vi "UpdateClassTemplate.vi"(0 "ClassWriterGOOP300In":refnum<class "ClassWriterGOOP300.lvclass">, 1 "LVClassLibraryRef":refnum<vi>, 2 "ProgressBar":refnum<vi>, 5 "error in (no error)":errorcluster) -> (14 "ClassWriterGOOP300Out":refnum<class "ClassWriterGOOP300.lvclass">, 19 "error out":errorcluster)   [LabVIEW 2016, in "ClassWriterGOOP300.lvclass"]
uses:
  <resource>/Framework/Providers/Open_GDS/ClassProviders/Provider_EndevoGOOP300/ClassWriterGOOP300_class/ClassWriterGOOP300.lvclass
  <resource>/Framework/Providers/Open_GDS/ClassProviders/Common/ScriptingFunctions/Scripting.lvclass
  <resource>/Framework/Providers/Open_GDS/ClassProviders/Provider_LvNativeClass/ClassWriterNative_class/ClassWriterNative.lvclass
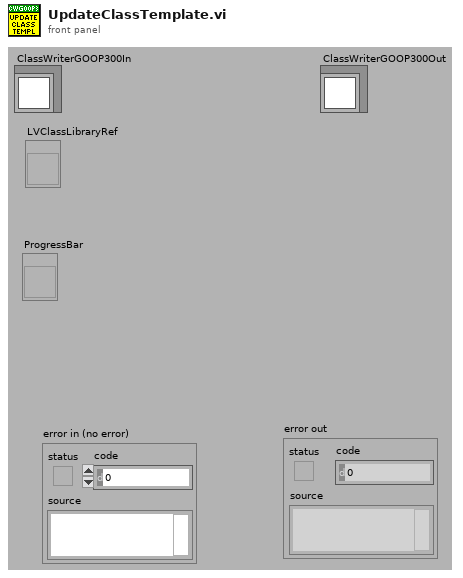
[diagram p1: front panel]
types:
  T1 = cluster{"VIs":refnum<vi>[], "VIRelPath":path[], "Application":refnum<vi>, "TemplateVersions":string, "Create":refnum<vi>, "NewVIIdx":i32}
  T2 = enum32{"invalid lock state", "Not Locked", "Locked (No Password)", "Password-protected"}
  T3 = enum16{"Share clones between instances", "Preallocate clone for each instance"}
  T4 = typedef "Scripting.lvclass/Scripting_PastThroughObjectType.ctl" = cluster{"Object":refnum<vi>, "InsideArray":bool, "PastThroughObjectTypes":T5[], "ObjectType":string, "ObjectData":string}
  T5 = typedef "Scripting_ObjectType.ctl" = cluster{"ObjectType":string, "ObjectName":string, "ObjectTerminalName":string}
  T6 = typedef "GDSLvCLass_ClassSettingsType.ctl" = cluster{"ClassProviderName":string, "ClassTemplateUsed":string, "ClassTemplateVersion":string, "ClassDescription":string, "PlugIns":T7[], "ConnectorPanePattern":string}
  T7 = typedef "GDSLvClass_PlugIn.ctl" = cluster{"Type":T8, "ID":string, "Version":string, "Path":path, "Name":string, "Data":variant}
  T8 = typedef "GDSLvClass_PlugInTypes.ctl" = enum16{"DesignPattern", "MethodTypes"}
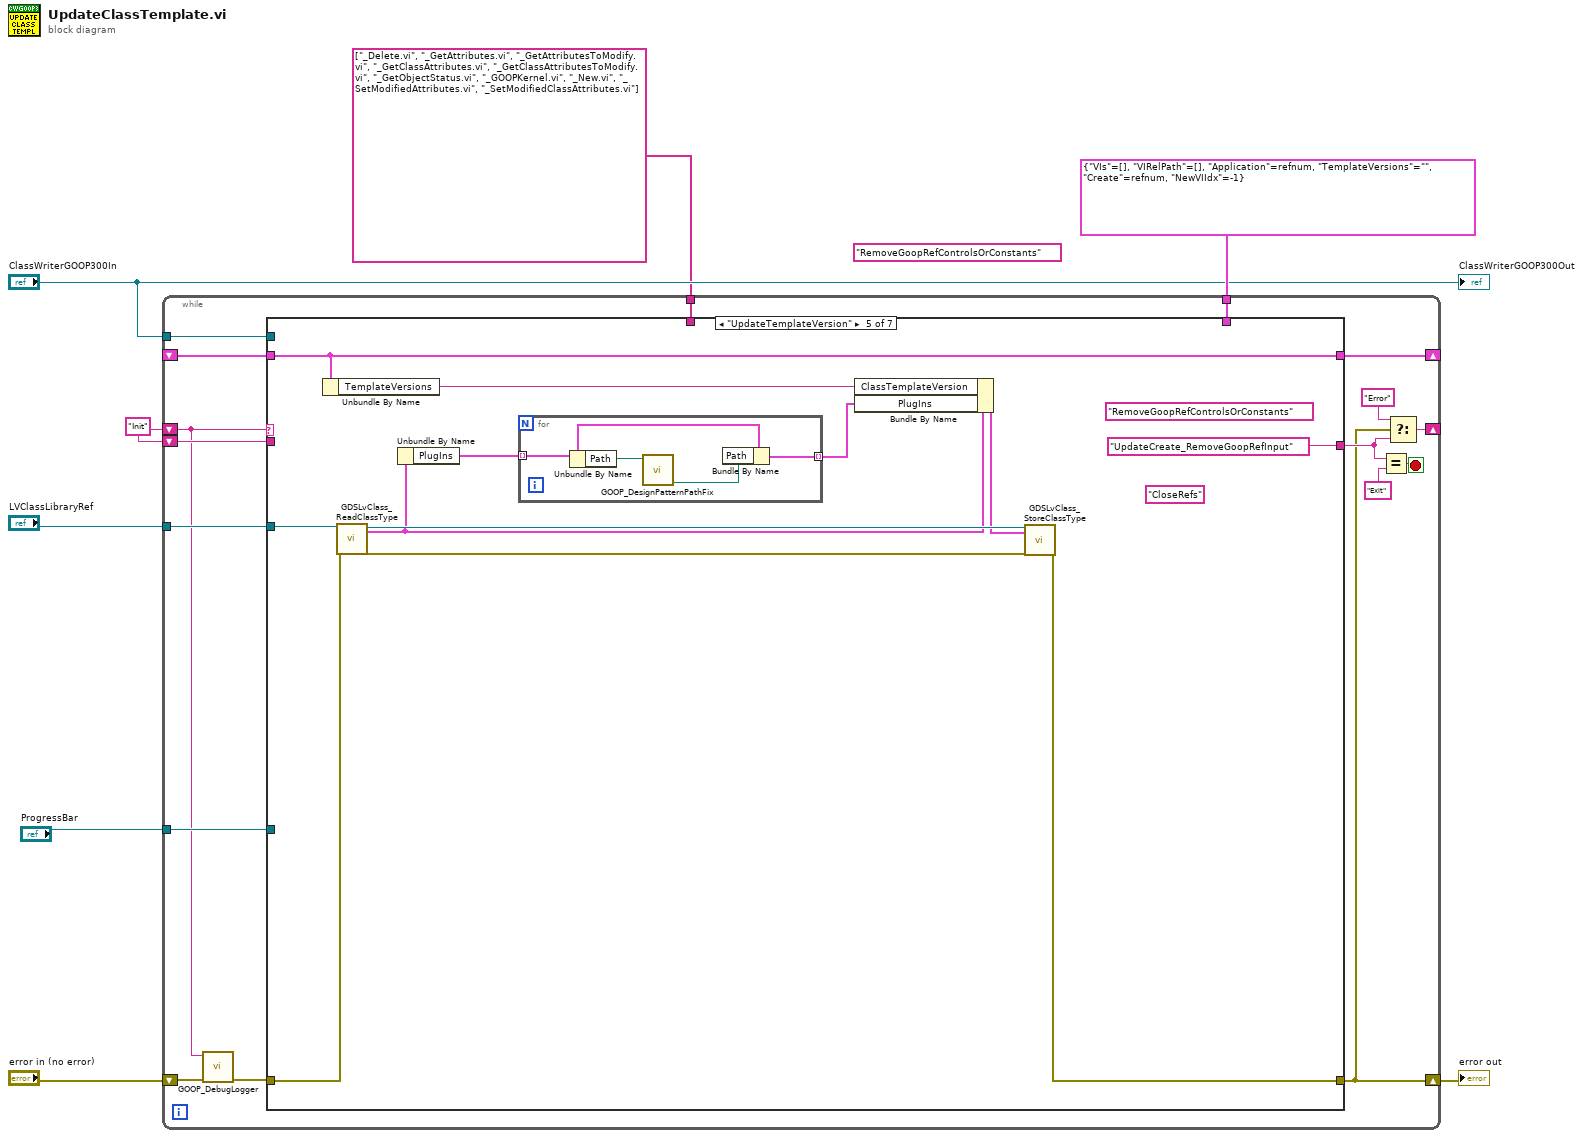
[diagram p0: block diagram]
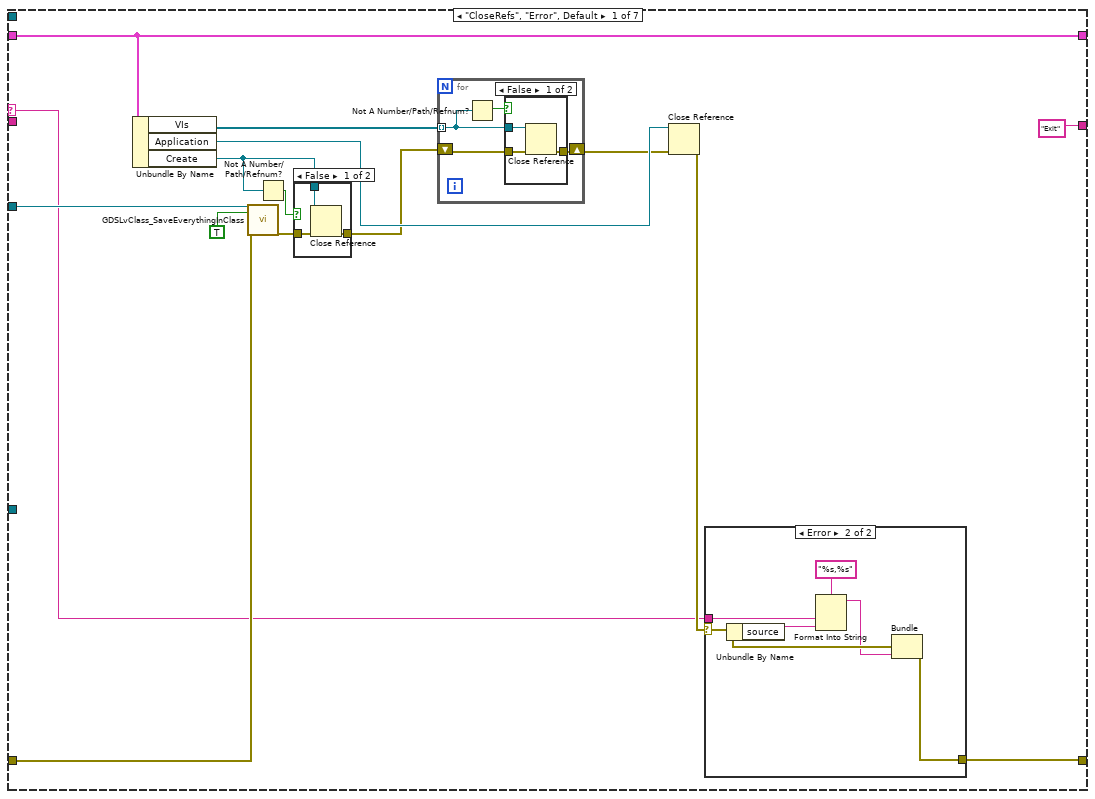
[diagram p2: hidden frame]
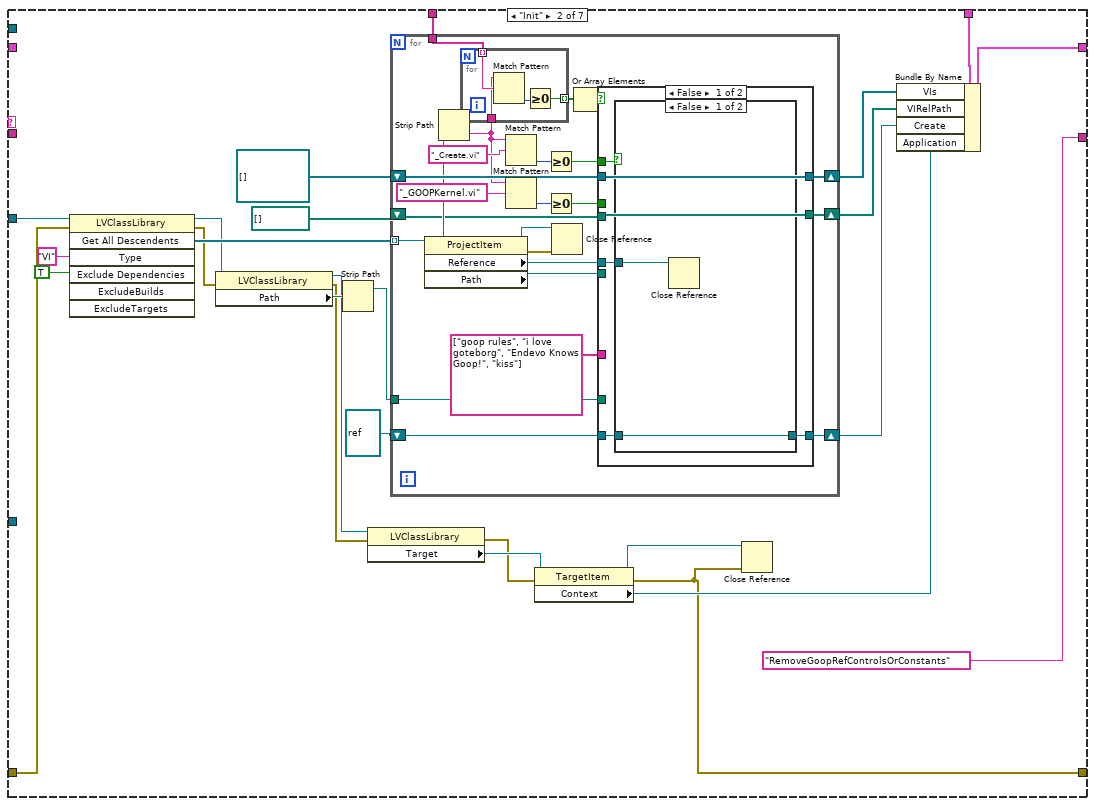
[diagram p6: hidden frame]
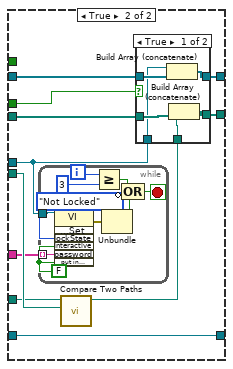
[diagram p8: hidden frame]
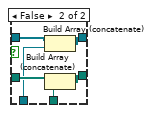
[diagram p9: hidden frame]
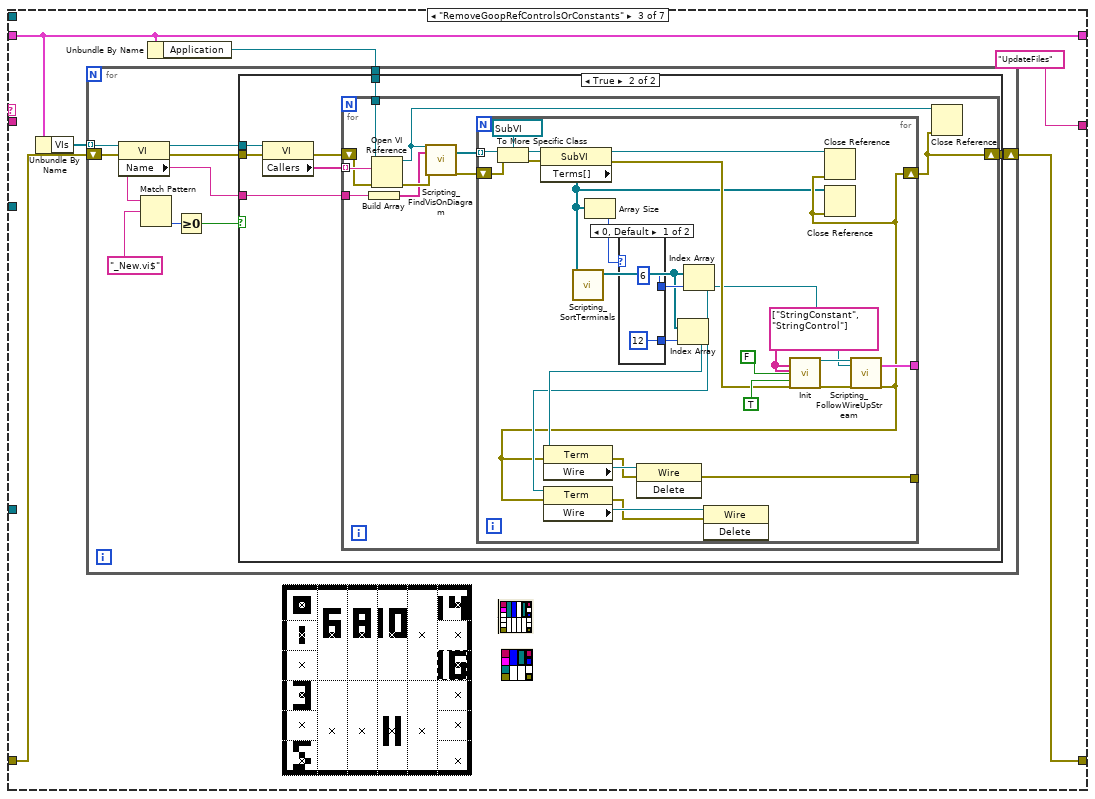
[diagram p10: hidden frame]
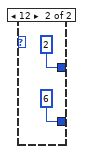
[diagram p12: hidden frame]
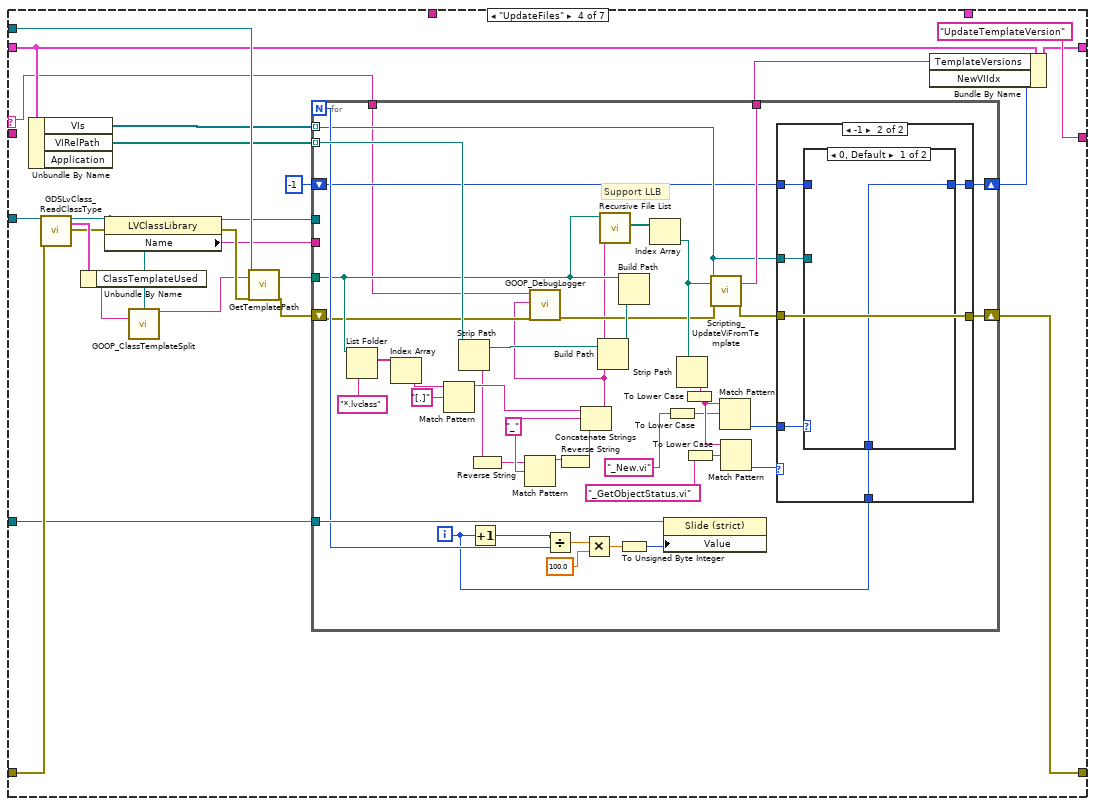
[diagram p13: hidden frame]
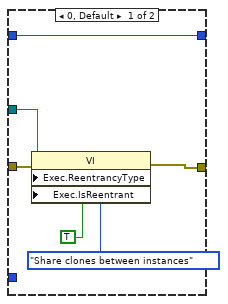
[diagram p14: hidden frame]
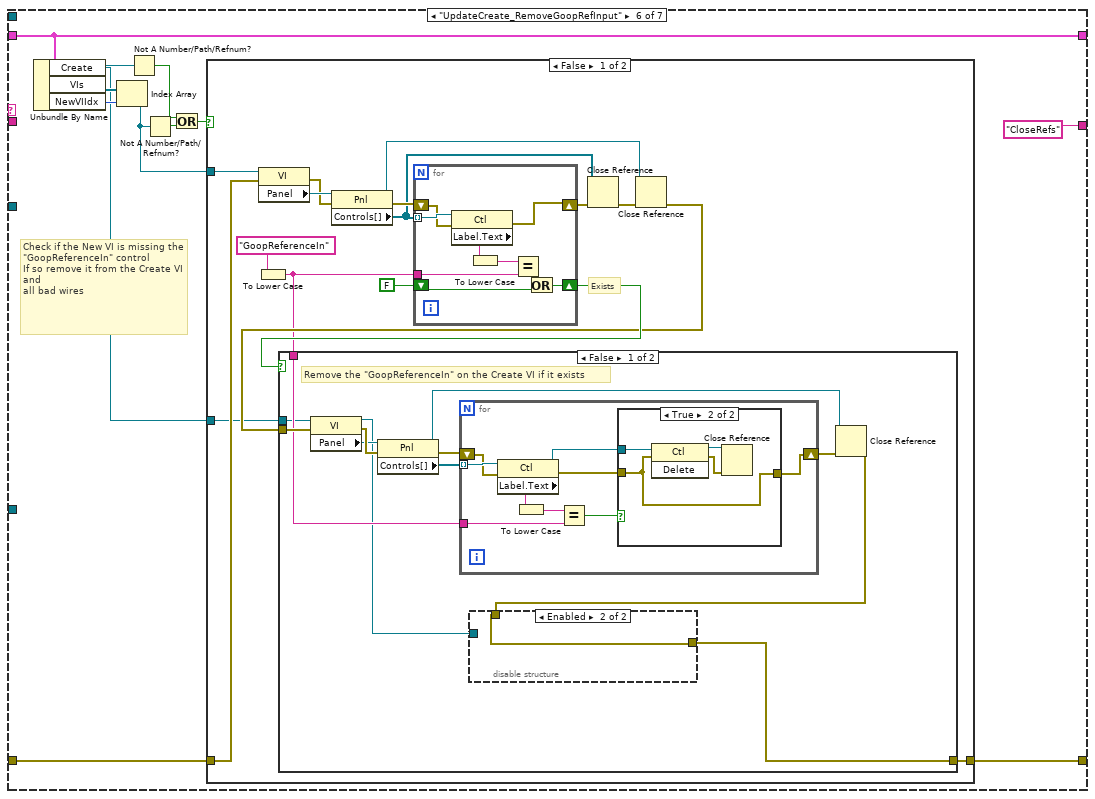
[diagram p16: hidden frame]
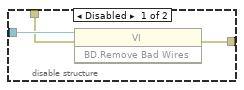
[diagram p17: hidden frame]
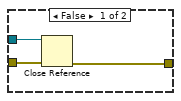
[diagram p18: hidden frame]
diagram:
  (unwired) "RemoveGoopRefControlsOrConstants"
  w1 = "Init"
  n1 = while {
    shift-right: [w20] -> w7
    shift-left: "error in (no error)" -> [w11]
    shift-right: [w25] -> _
    shift-left: w1 -> [w9]
    shift-right: [w19] -> _
    shift-left: _ -> [w18]
    tunnel: "LVClassLibraryRef" -> [w17]
    tunnel: T1 {"VIs"=[], "VIRelPath"=[], "Application"=refnum, "TemplateVersions"="", "Create"=refnum, "NewVIIdx"=-1} -> [w16]
    tunnel: "ClassWriterGOOP300In" -> [w15]
    tunnel: "ProgressBar" -> [w14]
    tunnel: string[] ["_Delete.vi", "_GetAttributes.vi", "_GetAttributesToModify.vi", "_GetClassAttributes.vi", "_GetClassAttributesToModify.vi", "_GetObjectStatus.vi", "_GOOPKernel.vi", "_New.vi", "_SetModifiedAttributes.vi", "_SetModifiedClassAttributes.vi"] ("Array") -> [w13]
    shift-left: w1 -> [w12]
    stop <- w24 stop-if-true
    n2 = call <resource>:"GOOP_DebugLogger.vi"("error in (no error)"=w11, "State"=w9) -> ("error out"=w10:errorcluster)  [unwired: 7 in, 2 out]
    n3 = case shown="\"UpdateTemplateVersion\"" w9 {
      selector: w9 -> [w28 _ _ w222 _ _ _]
      tunnel: w10 -> [w34 w66 w157 w234 w302 w317 w386]
      tunnel: [w27 w61 w159 w227 w301 w316 w386] -> w20
      tunnel: ["Exit" "RemoveGoopRefControlsOrConstants" "UpdateFiles" "UpdateTemplateVersion" "UpdateCreate_RemoveGoopRefInput" "CloseRefs" "Exit"] -> w21
      tunnel: [w39 w85 w156 w229 w308 w323 w385] -> w19
      tunnel: w18 -> [w39 _ w156 w230 w308 w323 w385]
      tunnel: w17 -> [w35 w84 _ w241 w307 _ _]
      tunnel: w16 -> [_ w78 _ _ _ _ _]
      tunnel: w15 -> [_ _ _ w239 _ _ _]
      tunnel: w14 -> [_ _ _ w226 _ _ _]
      tunnel: w13 -> [_ w65 _ _ _ _ _]
      tunnel: w12 -> [_ _ _ _ _ _ _]
      frame "CloseRefs", "Error", Default {
        n4 = Unbundle By Name(w39) -> ("VIs"=w38:refnum<vi>[], "Application"=w37:refnum<vi>, "Create"=w31:refnum<vi>)
        n5 = call <resource>:"GDSLvClass_SaveEverythingInClass.vi"("ClassRefIn"=w35, "ForceResaving(False)"=TRUE, "error in"=w34) -> ("error out"=w33:errorcluster)  [unwired: 15 in, 1 out]
        n6 = Not A Number/Path/Refnum?(number/path/refnum=w31) -> (NaN/Path/Refnum?=w30:bool)
        n7 = case shown="False" w30 {
          tunnel: w33 -> [w50 w51]
          tunnel: [w49 w51] -> w32
          tunnel: w31 -> [w48 _]
          frame False {
            n8 = Close Reference(reference=w48, error in (no error)=w50) -> (error out=w49:errorcluster)
          }
          frame True {
          }
        }
        n9 = for {
          tunnel: w38 -> [w53] mode=indexing
          shift-right: [w54] -> w26
          shift-left: w32 -> [w55]
          n10 = Not A Number/Path/Refnum?(number/path/refnum=w53) -> (NaN/Path/Refnum?=w52:bool)
          n11 = case shown="False" w52 {
            tunnel: w55 -> [w58 w59]
            tunnel: [w57 w59] -> w54
            tunnel: w53 -> [w56 _]
            frame False {
              n12 = Close Reference(reference=w56, error in (no error)=w58) -> (error out=w57:errorcluster)
            }
            frame True {
            }
          }
        }
        n13 = Close Reference(reference=w37, error in (no error)=w26) -> (error out=w29:errorcluster)
        n14 = case shown="Error" w29 {
          selector: w29 -> [w41 w44]
          tunnel: w28 -> [_ w46]
          tunnel: [w41 w42] -> w27
          frame No Error {
          }
          frame Error {
            n15 = Unbundle By Name(w44) -> ("source"=w45:string)
            n16 = Format Into String(format string="%s,%s", w46, w45) -> (resulting string=w43:string)  [unwired: 2 in, 1 out]
            n17 = Bundle(cluster=w44, "source"=w43) -> (w42:errorcluster)  [unwired: 2 in]
          }
        }
      }
      frame "Init" {
        n18 = invoke class="LVClassLibrary" method="Get All Descendents"(reference=w84, error in=w66, "Type"="VI", "Exclude Dependencies"=TRUE ("ExcludeDependencies")) -> (reference out=w80:refnum<vi>, error out=w69:errorcluster, "All Descendents"=w81:refnum<vi>[])  [unwired: 3 in, 4 out]
        n19 = property class="LVClassLibrary"(reference=w80, error in=w69) -> (reference out=w73:refnum<vi>, error out=w70:errorcluster, "Path"=w76:path)
        n20 = Strip Path(path=w76) -> (stripped path=w75:path)  [unwired: 1 out]
        n21 = property class="LVClassLibrary"(reference=w73, error in=w70) -> (error out=w71:errorcluster, "Target"=w72:refnum<vi>)  [unwired: 1 out]
        n22 = for {
          tunnel: w81 -> [w108] mode=indexing
          shift-right: [w106] -> w77
          shift-left: refnum<vi>[] [] -> [w107]
          shift-right: [w102] -> w68
          shift-left: path[] [] -> [w103]
          tunnel: w75 -> [w104]
          tunnel: w65 -> [w95]
          shift-right: [w91] -> w63
          shift-left: refnum<vi> refnum ("Reference") -> [w90]
          n23 = property class="ProjectItem"(reference=w108) -> (reference out=w99:refnum<vi>, error out=w101:errorcluster, "Reference"=w100:refnum<vi>, "Path"=w105:path)  [unwired: 1 in]
          n24 = Strip Path(path=w105) -> (name=w89:string)  [unwired: 1 out]
          n25 = for {
            tunnel: w95 -> [w112] mode=indexing
            tunnel: [w110] -> w97 mode=indexing
            tunnel: w89 -> [w109]
            n26 = Match Pattern(string=w109, regular expression=w112) -> (offset past match=w111:i32)  [unwired: 1 in, 3 out]
            n27 = Greater Or Equal To 0?(x=w111) -> (x >= 0?=w110:bool)
          }
          n28 = Match Pattern(string=w89, regular expression="_Create.vi") -> (offset past match=w93:i32)  [unwired: 1 in, 3 out]
          n29 = Match Pattern(string=w89, regular expression="_GOOPKernel.vi") -> (offset past match=w88:i32)  [unwired: 1 in, 3 out]
          n30 = Greater Or Equal To 0?(x=w93) -> (x >= 0?=w92:bool)
          n31 = Greater Or Equal To 0?(x=w88) -> (x >= 0?=w86:bool)
          n32 = Close Reference(reference=w99, error in (no error)=w101) -> ()  [unwired: 1 out]
          n33 = Or Array Elements(Boolean array=w97) -> (logical OR=w96:bool)
          n34 = case shown="False" w96 {
            tunnel: w107 -> [w118 w132]
            tunnel: w100 -> [w114 w125]
            tunnel: [w118 w131] -> w106
            tunnel: w105 -> [_ w127]
            tunnel: w104 -> [_ w126]
            tunnel: w103 -> [w117 w130]
            tunnel: [w117 w129] -> w102
            tunnel: string[] ["goop rules", "i love goteborg", "Endevo Knows Goop!", "kiss"] -> [_ w124]
            tunnel: w92 -> [w116 _]
            tunnel: [w115 w123] -> w91
            tunnel: w90 -> [w113 w123]
            tunnel: w86 -> [_ w122]
            frame False {
              n35 = case shown="False" w116 {
                tunnel: [w119 w121] -> w115
                tunnel: w114 -> [w120 w121]
                tunnel: w113 -> [w119 _]
                frame False {
                  n36 = Close Reference(reference=w120) -> ()  [unwired: 1 in, 1 out]
                }
                frame True {
                }
              }
            }
            frame True {
              n37 = while {
                tunnel: w125 -> [w152]
                tunnel: w124 -> [w151] mode=indexing
                i -> [w148]
                stop <- w149 stop-if-true
                w153 = FALSE ("Interactive")
                n38 = invoke class="VI" method="Lock State.Set"(reference=w152, "lockState"=T2."Not Locked" ("Lock State"), "interactive"=w153, "password"=w151, "put in Cache"=w153) -> (error out=w150:errorcluster)  [unwired: 2 in, 6 out]
                n39 = Greater Or Equal?(x=w148, y=3) -> (x >= y?=w147:bool)
                n40 = Unbundle(w150) -> ("status"=w145:bool)  [unwired: 2 out]
                n41 = Compound Arithmetic op=OR(w147, invert w145) -> (w149:bool)
              }
              n42 = call <vilib>:"Compare Two Paths.vi"("Path 2"=w127, "Path 1"=w126) -> ("Relative Path from 1 to 2"=w128:path)  [unwired: 6 in, 3 out]
              n43 = case shown="True" w122 {
                tunnel: w132 -> [w138 w144]
                tunnel: [w137 w143] -> w131
                tunnel: w130 -> [w136 w142]
                tunnel: [w135 w141] -> w129
                tunnel: w128 -> [w134 w140]
                tunnel: w125 -> [w133 w139]
                frame True {
                  n44 = Build Array (concatenate)(w133, w138) -> (w137:refnum<vi>[])
                  n45 = Build Array (concatenate)(w134, w136) -> (w135:path[])
                }
                frame False {
                  n46 = Build Array (concatenate)(w144, w139) -> (w143:refnum<vi>[])
                  n47 = Build Array (concatenate)(w142, w140) -> (w141:path[])
                }
              }
            }
          }
        }
        n48 = property class="TargetItem"(reference=w72, error in=w71) -> (reference out=w60:refnum<vi>, error out=w61:errorcluster, "Context"=w67:refnum<vi>)
        n49 = Close Reference(reference=w60, error in (no error)=w61) -> ()  [unwired: 1 out]
        n50 = Bundle By Name(cluster=w78, "VIs"=w77, "VIRelPath"=w68, "Create"=w63, "Application"=w67) -> (w85:T1)
      }
      frame "RemoveGoopRefControlsOrConstants" {
        n51 = Unbundle By Name(w156) -> ("VIs"=w160:refnum<vi>[])
        n52 = Unbundle By Name(w156) -> ("Application"=w155:refnum<vi>)
        n53 = for {
          tunnel: w160 -> [w169] mode=indexing
          shift-right: [w170] -> w159
          shift-left: w157 -> [w168]
          tunnel: w155 -> [w161]
          n54 = property class="VI"(reference=w169, error in=w168) -> (reference out=w164:refnum<vi>, error out=w163:errorcluster, "Name"=w162:string)
          n55 = Match Pattern(string=w162, regular expression="_New.vi$") -> (offset past match=w166:i32)  [unwired: 1 in, 3 out]
          n56 = Greater Or Equal To 0?(x=w166) -> (x >= 0?=w165:bool)
          n57 = case shown="True" w165 {
            tunnel: w164 -> [_ w177]
            tunnel: w163 -> [w171 w174]
            tunnel: [w171 w178] -> w170
            tunnel: w162 -> [_ w173]
            tunnel: w161 -> [_ w172]
            frame False {
            }
            frame True {
              n58 = property class="VI"(reference=w177, error in=w174) -> (error out=w175:errorcluster, "Callers"=w176:string[])  [unwired: 1 out]
              n59 = for {
                tunnel: w176 -> [w186] mode=indexing
                tunnel: w173 -> [w184]
                shift-right: [w180] -> w178
                shift-left: w175 -> [w185]
                tunnel: w172 -> [w181]
                n60 = Build Array(w184) -> (w182:string[])
                n61 = Open VI Reference(application reference (local)=w181, vi path=w186, error in (no error)=w185) -> (vi reference=w179:refnum<vi>, error out=w183:errorcluster)  [unwired: 3 in]
                n62 = call <resource>:"Scripting_FindVisOnDiagram.vi"("ViRef"=w179, "VIsToSerachFor/ViName"=w182, "error in (no error)"=w183) -> ("VisFound"=w188:refnum<vi>[], "error out"=w187:errorcluster)  [unwired: 15 in]
                n63 = for {
                  tunnel: w188 -> [w213] mode=indexing
                  shift-right: [w190] -> w180
                  shift-left: w187 -> [w212]
                  tunnel: [w202] -> _
                  tunnel: [w194] -> _
                  w206 = string[] ["StringConstant", "StringControl"] ("FindAnyOfTheseClassTypes")
                  n64 = To More Specific Class(target class=refnum<vi> refnum ("WhileLoop"), reference=w213, error in=w212) -> (specific class reference=w211:refnum<vi>, error out=w210:errorcluster)
                  n65 = property class="SubVI"(reference=w211, error in=w210) -> (reference out=w200:refnum<vi>, error out=w201:errorcluster, "Terms[]"=w189:refnum<vi>[])
                  n66 = call <resource>:"Scripting_SortTerminals.vi"("Terminals[]"=w189) -> ("TerminalsOut[]"=w199:refnum<vi>[])  [unwired: 8 in, 2 out]
                  n67 = Array Size(array=w189) -> (size(s)=w205:i32)
                  n68 = case shown="0, Default" w205 {
                    tunnel: [6 ("index") 2 ("index")] -> w204
                    tunnel: [12 ("index") 6 ("index")] -> w198
                    frame 0, Default {
                    }
                    frame 12 {
                    }
                  }
                  n69 = Index Array(array=w199, index=w198) -> (element=w197:refnum<vi>)
                  n70 = Index Array(array=w199, index=w204) -> (element=w193:refnum<vi>)
                  n71 = call <resource>:"Init.vi"("FindAnyOfTheseClassTypes"=w206, "StopWhenAnyOfTheseClassTypesAreReached"=w206, "KeepObjectsOpen(True)"=FALSE, "DeleteWires(False)"=TRUE ("KeepObjectsOpen(True)"), "error in (no error)"=w201) -> ("object out"=w208:refnum<class "Scripting.lvclass">, "error out"=w209:errorcluster)  [unwired: 13 in]
                  n72 = call-dynamic "Scripting_FollowWireUpStream.vi"("Scripting in"=w208, "StartTerminalRef"=w193, "error in (no error)"=w209) -> ("FoundItems"=w202:T4[], "error out"=w190:errorcluster)  [unwired: 15 in]
                  n73 = property class="Term"(reference=w197, error in=w190) -> (error out=w195:errorcluster, "Wire"=w196:refnum<vi>)  [unwired: 1 out]
                  n74 = property class="Term"(reference=w193, error in=w190) -> (error out=w191:errorcluster, "Wire"=w192:refnum<vi>)  [unwired: 1 out]
                  n75 = invoke class="Wire" method="Delete"(reference=w196, error in=w195) -> (error out=w194:errorcluster)  [unwired: 1 in, 2 out]
                  n76 = invoke class="Wire" method="Delete"(reference=w192, error in=w191) -> ()  [unwired: 1 in, 3 out]
                  n77 = Close Reference(reference=w200, error in (no error)=w190) -> ()  [unwired: 1 out]
                  n78 = Close Reference(reference=w189, error in (no error)=w190) -> ()  [unwired: 1 out]
                }
                n79 = Close Reference(reference=w179, error in (no error)=w180) -> ()  [unwired: 1 out]
              }
            }
          }
        }
      }
      frame "UpdateFiles" {
        n80 = Unbundle By Name(w230) -> ("VIs"=w236:refnum<vi>[], "VIRelPath"=w237:path[])  [unwired: 1 out]
        n81 = call <resource>:"GDSLvClass_ReadClassType.vi"("Class Refnum In"=w241, "error in (no error)"=w234) -> ("Class Refnum Out"=w219:refnum<vi>, "ClassSettings"=w240:T6, "error out"=w233:errorcluster)  [unwired: 15 in]
        n82 = Unbundle By Name(w240) -> ("ClassTemplateUsed"=w221:string)
        n83 = property class="LVClassLibrary"(reference=w219, error in=w233) -> (reference out=w225:refnum<vi>, error out=w232:errorcluster, "Name"=w231:string)
        n84 = call <resource>:"GOOP_ClassTemplateSplit.vi"("ClassItemRefIn"=w219, "FullClassTemplate"=w221) -> ("StandardTemplate"=w220:string)  [unwired: 12 in, 1 out]
        n85 = call-dynamic "GetTemplatePath.vi"("reference in"=w239, "ClassTemplateSubDirectory"=w220, "error in (no error)"=w232) -> ("FolderPathOut"=w238:path, "error out"=w235:errorcluster)  [unwired: 12 in, 3 out]
        n86 = for {
          N -> [w264]
          tunnel: w238 -> [w262]
          tunnel: w237 -> [w279] mode=indexing
          tunnel: w236 -> [w254] mode=indexing
          shift-right: [w255] -> w227
          shift-left: w235 -> [w246]
          tunnel: w231 -> [_]
          tunnel: [w270] -> w228
          tunnel: w226 -> [w266]
          tunnel: w225 -> [_]
          shift-right: [w251] -> w223
          shift-left: -1 -> [w250]
          tunnel: w222 -> [w244]
          i -> [w249]
          w283 = "_" ("regular expression")
          # "Support LLB"
          n87 = List Folder(path=w262, pattern="*.lvclass") -> (filenames=w275:string[])  [unwired: 2 in, 3 out]
          n88 = Index Array(array=w275) -> (element=w274:string)  [unwired: 1 in]
          n89 = Match Pattern(string=w274, regular expression="[.]") -> (before substring=w272:string)  [unwired: 1 in, 3 out]
          n90 = Strip Path(path=w279) -> (stripped path=w278:path, name=w271:string)
          n91 = Increment(x=w249) -> (x+1=w265:i32)
          n92 = Reverse String(1:w271) -> (0:w282:string)
          n93 = Match Pattern(string=w282, regular expression=w283) -> (before substring=w281:string)  [unwired: 1 in, 3 out]
          n94 = Divide(x=w265, y=w264) -> (x/y=w269:dbl)
          n95 = Reverse String(1:w281) -> (0:w280:string)
          n96 = Concatenate Strings(w272, w283, w280) -> (w243:string)
          n97 = call <resource>:"GOOP_DebugLogger.vi"("error in (no error)"=w246, "Data"=w243, "State"=w244) -> ("error out"=w245:errorcluster)  [unwired: 6 in, 2 out]
          n98 = Multiply(x=w269, y=100.0) -> (x*y=w267:dbl)
          n99 = Build Path(base path=w278, name or relative path=w243) -> (appended path=w277:path)
          n100 = call <vilib>:"Recursive File List.vi"("pattern"=w243, "Folder Path"=w262) -> ("All Files in Dir"=w261:path[])  [unwired: 5 in, 4 out]
          n101 = Build Path(base path=w262, name or relative path=w277) -> ()  [unwired: 1 out]
          n102 = To Unsigned Byte Integer(number=w267) -> (unsigned 8bit integer=w263:u8)
          n103 = Index Array(array=w261) -> (element=w260:path)  [unwired: 1 in]
          n104 = property class="Slide (strict)"(reference=w266, "Value"=w263) -> ()  [unwired: 1 in, 2 out]
          n105 = To Lower Case(string="_New.vi" ("regular expression")) -> (all lower case string=w247:string)
          n106 = Strip Path(path=w260) -> (name=w259:string)  [unwired: 1 out]
          n107 = To Lower Case(string=w259) -> (all lower case string=w253:string)
          n108 = To Lower Case(string="_GetObjectStatus.vi" ("regular expression")) -> (all lower case string=w257:string)
          n109 = call <resource>:"Scripting_UpdateViFromTemplate.vi"("ViRef"=w254, "TemplateVI(Path or Ref)"=w260, "error in (no error)"=w245) -> ("TemplateVersionUsed"=w270:string, "error out"=w255:errorcluster)  [unwired: 15 in]
          n110 = Match Pattern(string=w253, regular expression=w247) -> (offset past match=w252:i32)  [unwired: 1 in, 3 out]
          n111 = Match Pattern(string=w253, regular expression=w257) -> (offset past match=w256:i32)  [unwired: 1 in, 3 out]
          n112 = case shown="-1" w256 {
            tunnel: w255 -> [w289 w295]
            tunnel: w254 -> [w288 w292]
            tunnel: [w285 w295] -> _
            tunnel: w252 -> [_ w294]
            tunnel: [w284 w293] -> w251
            tunnel: w250 -> [w284 w291]
            tunnel: w249 -> [_ w290]
            frame 0, Default {
              n113 = property class="VI"(reference=w288, error in=w289, "Exec.ReentrancyType"=T3."Share clones between instances" ("Execution:Reentrancy Type"), "Exec.IsReentrant"=TRUE ("Execution:Is Reentrant")) -> (error out=w285:errorcluster)  [unwired: 1 out]
            }
            frame -1 {
              n114 = case shown="0, Default" w294 {
                tunnel: [w296 w297] -> w293
                tunnel: w292 -> [_ _]
                tunnel: w291 -> [_ w297]
                tunnel: w290 -> [w296 _]
                frame 0, Default {
                }
                frame -1 {
                }
              }
            }
          }
        }
        n115 = Bundle By Name(cluster=w230, "TemplateVersions"=w228, "NewVIIdx"=w223) -> (w229:T1)
      }
      frame "UpdateTemplateVersion" {
        (unwired) "RemoveGoopRefControlsOrConstants"
        (unwired) "CloseRefs"
        n116 = Unbundle By Name(w308) -> ("TemplateVersions"=w303:string)
        n117 = call <resource>:"GDSLvClass_ReadClassType.vi"("Class Refnum In"=w307, "error in (no error)"=w302) -> ("Class Refnum Out"=w306:refnum<vi>, "ClassSettings"=w300:T6, "error out"=w305:errorcluster)  [unwired: 15 in]
        n118 = Unbundle By Name(w300) -> ("PlugIns"=w299:T7[])
        n119 = for {
          tunnel: w299 -> [w312] mode=indexing
          tunnel: [w310] -> w298 mode=indexing
          n120 = Unbundle By Name(w312) -> ("Path"=w313:path)
          n121 = call <resource>:"GOOP_DesignPatternPathFix.vi"("ViPathIn"=w313) -> ("RelativeVIPathOut(ToStoreInLvClass)"=w311:path)  [unwired: 6 in, 4 out]
          n122 = Bundle By Name(cluster=w312, "Path"=w311) -> (w310:T7)
        }
        n123 = Bundle By Name(cluster=w300, "ClassTemplateVersion"=w303, "PlugIns"=w298) -> (w304:T6)
        n124 = call <resource>:"GDSLvClass_StoreClassType.vi"("Class Refnum In"=w306, "ClassSettings"=w304, "error in (no error)"=w305) -> ("error out"=w301:errorcluster)  [unwired: 15 in, 1 out]
      }
      frame "UpdateCreate_RemoveGoopRefInput" {
        # "Check if the New VI is missing the\n\"GoopReferenceIn\" control\nIf so remove it from the Create VI and\nall bad wires"
        n125 = Unbundle By Name(w323) -> ("Create"=w314:refnum<vi>, "VIs"=w322:refnum<vi>[], "NewVIIdx"=w321:i32)
        n126 = Index Array(array=w322, index=w321) -> (element=w315:refnum<vi>)
        n127 = Not A Number/Path/Refnum?(number/path/refnum=w314) -> (NaN/Path/Refnum?=w320:bool)
        n128 = Not A Number/Path/Refnum?(number/path/refnum=w315) -> (NaN/Path/Refnum?=w319:bool)
        n129 = Or(x=w320, y=w319) -> (x .or. y?=w318:bool)
        n130 = case shown="False" w318 {
          tunnel: w317 -> [w330 w383]
          tunnel: [w326 w383] -> w316
          tunnel: w315 -> [w340 _]
          tunnel: w314 -> [w325 _]
          frame False {
            # "Exists"
            n131 = To Lower Case(string="GoopReferenceIn" ("y")) -> (all lower case string=w327:string)
            n132 = property class="VI"(reference=w340, error in=w330) -> (error out=w331:errorcluster, "Panel"=w339:refnum<vi>)  [unwired: 1 out]
            n133 = property class="Pnl"(reference=w339, error in=w331) -> (reference out=w332:refnum<vi>, error out=w336:errorcluster, "Controls[]"=w334:refnum<vi>[])
            n134 = for {
              tunnel: w334 -> [w382] mode=indexing
              tunnel: w327 -> [w379]
              shift-right: [w377] -> w329
              shift-left: FALSE -> [w376]
              shift-right: [w374] -> w335
              shift-left: w336 -> [w375]
              n135 = property class="Ctl"(reference=w382, error in=w375) -> (error out=w374:errorcluster, "Label.Text"=w381:string)  [unwired: 1 out]
              n136 = To Lower Case(string=w381) -> (all lower case string=w380:string)
              n137 = Equal?(x=w380, y=w379) -> (x = y?=w378:bool)
              n138 = Or(x=w378, y=w376) -> (x .or. y?=w377:bool)
            }
            n139 = Close Reference(reference=w334, error in (no error)=w335) -> (error out=w333:errorcluster)
            n140 = Close Reference(reference=w332, error in (no error)=w333) -> (error out=w328:errorcluster)
            n141 = case shown="False" w329 {
              tunnel: w328 -> [w347 w373]
              tunnel: w327 -> [w346 _]
              tunnel: [w342 w373] -> w326
              tunnel: w325 -> [w341 _]
              frame False {
                # "Remove the \"GoopReferenceIn\" on the Create VI if it exists"
                n142 = property class="VI"(reference=w341, error in=w347) -> (reference out=w344:refnum<vi>, error out=w352:errorcluster, "Panel"=w348:refnum<vi>)
                n143 = property class="Pnl"(reference=w348, error in=w352) -> (reference out=w351:refnum<vi>, error out=w349:errorcluster, "Controls[]"=w350:refnum<vi>[])
                n144 = for {
                  tunnel: w350 -> [w365] mode=indexing
                  tunnel: w346 -> [w362]
                  shift-right: [w357] -> w345
                  shift-left: w349 -> [w361]
                  n145 = property class="Ctl"(reference=w365, error in=w361) -> (reference out=w358:refnum<vi>, error out=w359:errorcluster, "Label.Text"=w364:string)
                  n146 = To Lower Case(string=w364) -> (all lower case string=w363:string)
                  n147 = Equal?(x=w363, y=w362) -> (x = y?=w360:bool)
                  n148 = case shown="True" w360 {
                    tunnel: w359 -> [w368 w371]
                    tunnel: w358 -> [w367 w372]
                    tunnel: [w366 w371] -> w357
                    frame False {
                      n149 = Close Reference(reference=w367, error in (no error)=w368) -> (error out=w366:errorcluster)
                    }
                    frame True {
                      n150 = invoke class="Ctl" method="Delete"(reference=w372, error in=w371) -> (reference out=w370:refnum<vi>, error out=w369:errorcluster)  [unwired: 1 in, 1 out]
                      n151 = Close Reference(reference=w370, error in (no error)=w369) -> ()  [unwired: 1 out]
                    }
                  }
                }
                n152 = Close Reference(reference=w351, error in (no error)=w345) -> (error out=w343:errorcluster)
                n153 = disable-structure shown="Enabled" {
                  disable-tunnel: w344 -> [w355 _]
                  disable-tunnel: w343 -> [w354 w356]
                  disable-tunnel: [w353 w356] -> w342
                  frame Disabled {
                    n154 = invoke class="VI" method="BD.Remove Bad Wires"(reference=w355, error in=w354) -> (error out=w353:errorcluster)  [unwired: 1 in, 2 out]
                  }
                  frame Enabled {
                  }
                }
              }
              frame True {
                # "Don't do anything"
              }
            }
          }
          frame True {
          }
        }
      }
      frame "Idle" {
      }
    }
    n155 = Equal?(x=w21, y="Exit") -> (x = y?=w24:bool)
    n156 = Select(t="Error", s=w20, f=w21) -> (s? t:f=w25:string)
  }
  "error out" <- w7
  "ClassWriterGOOP300Out" <- "ClassWriterGOOP300In"
